vi "monitor.vi"() -> ()   [LabVIEW 2013]
uses:
  controler_custer.ctl
  <vilib>/Instr/_visa.llb/VISA Configure Serial Port (Instr).vi
panel:
  in  "Log folder":path=path "Y:/"
  in  "Sampling interval (s)":dbl=300.0
  out "DataFrontN":T1 {"Power" format="%.2g"; "Voltage" format="%.2g"; "Current" format="%.2g"; "Regulator" format="%.2g"; "Extra sensor" format="%.2g"; "Cold plate" format="%.2g"; "Set point" format="%.2g"; "Main sensor" format="%.2g"}
  in  "Input frontN":T2={"Port"="COM7", "Log file"="frontN.txt", "LogData"=TRUE}
  out "DataFrontS":T1 {"Power" format="%.2g"; "Voltage" format="%.2g"; "Current" format="%.2g"; "Regulator" format="%.2g"; "Extra sensor" format="%.2g"; "Cold plate" format="%.2g"; "Set point" format="%.2g"; "Main sensor" format="%.2g"}
  in  "Input frontS":T2={"Port"="COM6", "Log file"="frontS.txt", "LogData"=TRUE}
  out "DataBottomN":T1 {"Power" format="%.2g"; "Voltage" format="%.2g"; "Current" format="%.2g"; "Regulator" format="%.2g"; "Extra sensor" format="%.2g"; "Cold plate" format="%.2g"; "Set point" format="%.2g"; "Main sensor" format="%.2g"}
  in  "Input bottomN":T2={"Port"="COM11", "Log file"="bottomN.txt", "LogData"=TRUE}
  out "DataBottomS":T1 {"Power" format="%.2g"; "Voltage" format="%.2g"; "Current" format="%.2g"; "Regulator" format="%.2g"; "Extra sensor" format="%.2g"; "Cold plate" format="%.2g"; "Set point" format="%.2g"; "Main sensor" format="%.2g"}
  in  "Input bottomS":T2={"Port"="COM10", "Log file"="bottomS.txt", "LogData"=TRUE}
  out "DataTopN":T1 {"Power" format="%.2g"; "Voltage" format="%.2g"; "Current" format="%.2g"; "Regulator" format="%.2g"; "Extra sensor" format="%.2g"; "Cold plate" format="%.2g"; "Set point" format="%.2g"; "Main sensor" format="%.2g"}
  in  "Input topN":T3={"Port"="COM9", "Log file"="topN.txt", "logData"=TRUE}
  out "DataTopS":T1 {"Power" format="%.2g"; "Voltage" format="%.2g"; "Current" format="%.2g"; "Regulator" format="%.2g"; "Extra sensor" format="%.2g"; "Cold plate" format="%.2g"; "Set point" format="%.2g"; "Main sensor" format="%.2g"}
  in  "Input topS":T2={"Port"="COM8", "Log file"="topS.txt", "LogData"=TRUE}
  out "start time":timestamp
  in  "Connect all":bool
  in  "stop":bool
  # "Top S"
  # "Top N"
  # "Bottom S"
  # "Bottom N"
  # "Front S"
  # "Front N"
  # "Temeprature"
  # "Temeprature"
  # "Temeprature"
  # "Temeprature"
  # "Temeprature"
  # "Temeprature"
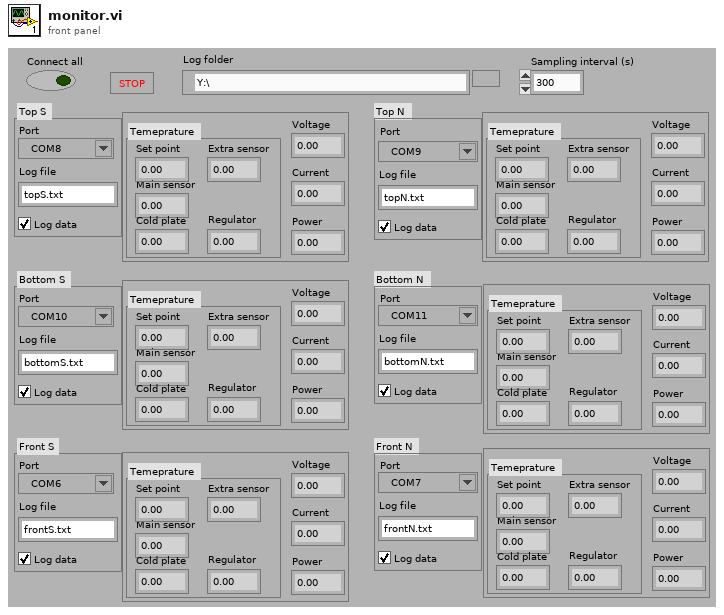
[diagram p1: front panel]
types:
  T1 = typedef "controler_custer.ctl" = cluster{"Set point":dbl, "Main sensor":dbl, "Cold plate":dbl, "Extra sensor":dbl, "Regulator":dbl, "Voltage":dbl, "Current":dbl, "Power":dbl}
  T2 = cluster{"Port":refnum<visa-resource-name>, "Log file":string, "LogData":bool}
  T3 = cluster{"Port":refnum<visa-resource-name>, "Log file":string, "logData":bool}
  T4 = cluster{"readSetPoint":string, "readT1":string, "readT2":string, "readT3":string, "readT4":string, "readV":string, "readI":string, "readPower":string}
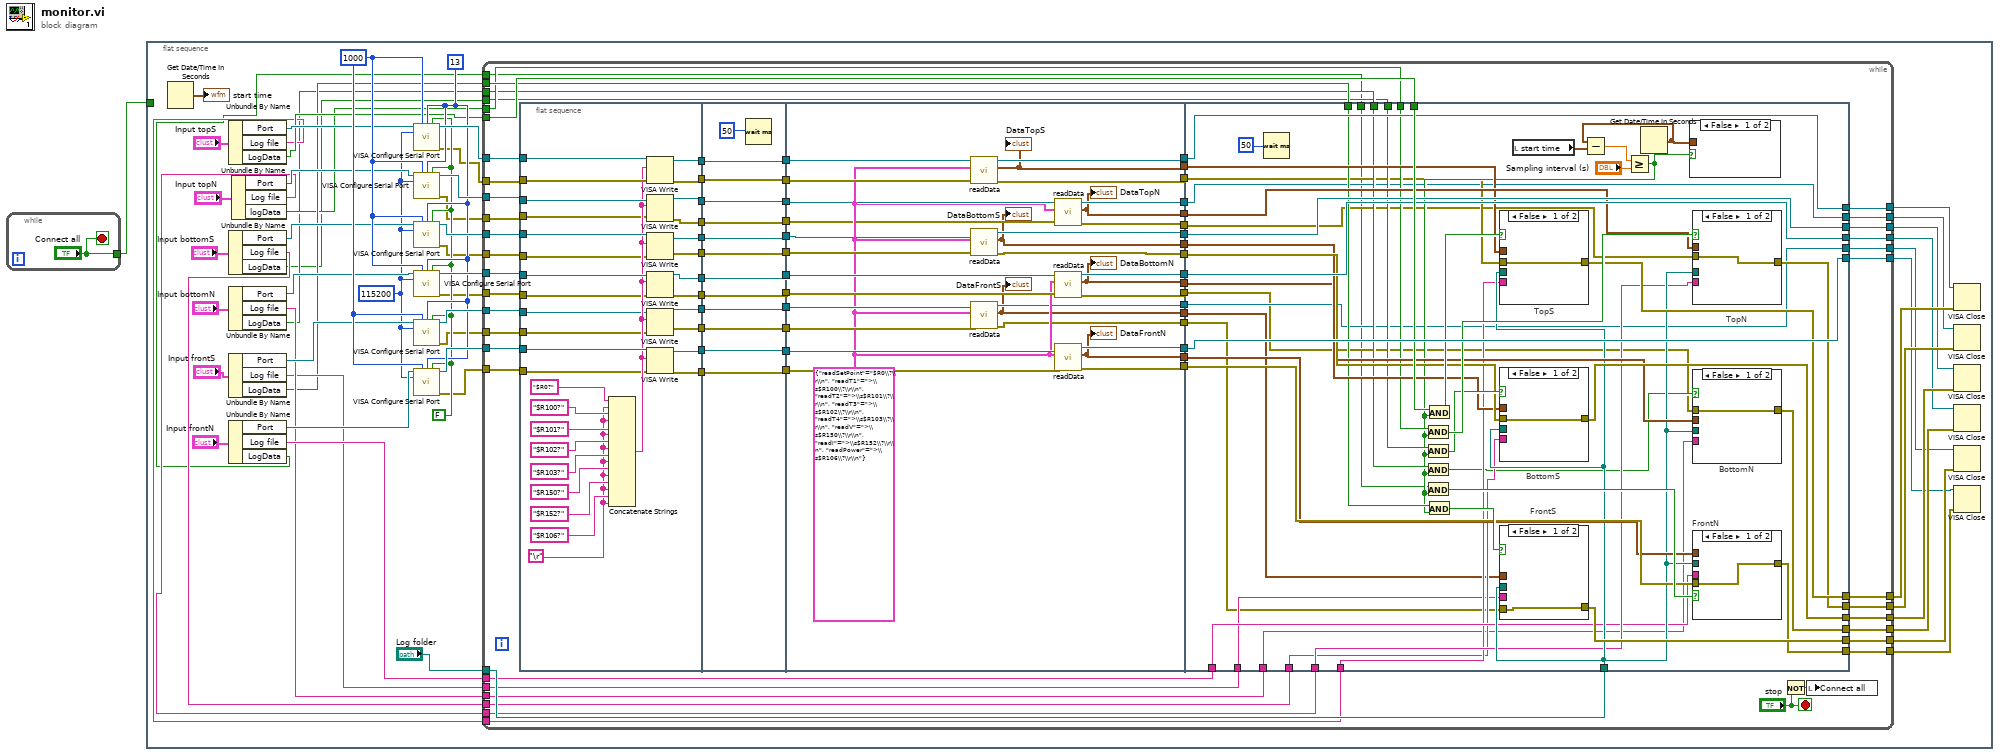
[diagram p0: block diagram]
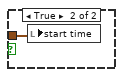
[diagram p2: hidden frame]
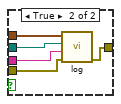
[diagram p3: hidden frame]
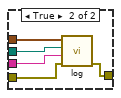
[diagram p4: hidden frame]
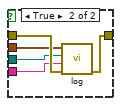
[diagram p5: hidden frame]
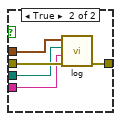
[diagram p6: hidden frame]
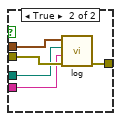
[diagram p7: hidden frame]
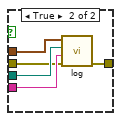
[diagram p8: hidden frame]
diagram:
  n1 = while {
    tunnel: ["Connect all"] -> w1
    stop <- "Connect all" stop-if-true
  }
  n2 = flat-sequence {
    tunnel: w1 -> [_]
    frame #0 {
      w10 = u32 115200 ("baud rate (9600)")
      w50 = u32 1000 ("timeout (10sec)")
      w48 = FALSE ("Enable Termination\nChar (T)")
      w49 = u8 13 ("termination char\n(0xA = '\\n' = LF)")
      n3 = Get Date/Time In Seconds() -> (seconds since 1Jan1904=→"start time":timestamp)
      n4 = Unbundle By Name("Input topS") -> ("Port"=w37:refnum<visa-resource-name>, "Log file"=w19:string, "LogData"=w36:bool)
      n5 = Unbundle By Name("Input bottomS") -> ("Port"=w29:refnum<visa-resource-name>, "Log file"=w18:string, "LogData"=w12:bool)
      n6 = Unbundle By Name("Input bottomN") -> ("Port"=w28:refnum<visa-resource-name>, "Log file"=w17:string, "LogData"=w13:bool)
      n7 = Unbundle By Name("Input frontS") -> ("Port"=w27:refnum<visa-resource-name>, "Log file"=w16:string, "LogData"=w15:bool)
      n8 = Unbundle By Name("Input frontN") -> ("Port"=w26:refnum<visa-resource-name>, "Log file"=w20:string, "LogData"=w11:bool)
      n9 = Unbundle By Name("Input topN") -> ("Port"=w30:refnum<visa-resource-name>, "Log file"=w21:string, "logData"=w14:bool)
      n10 = call-poly "VISA Configure Serial Port"("VISA resource name"=w37, "timeout (10sec)"=w50, "termination char\n(0xA = '\\n' = LF)"=w49, "Enable Termination\nChar (T)"=w48, "baud rate (9600)"=w10) -> ("VISA resource name out"=w56:refnum<visa-resource-name>, "error out"=w46:errorcluster)  [unwired: 9 in]
      n11 = call-poly "VISA Configure Serial Port"("VISA resource name"=w30, "timeout (10sec)"=w50, "termination char\n(0xA = '\\n' = LF)"=w49, "Enable Termination\nChar (T)"=w48, "baud rate (9600)"=w10) -> ("VISA resource name out"=w55:refnum<visa-resource-name>, "error out"=w45:errorcluster)  [unwired: 9 in]
      n12 = call-poly "VISA Configure Serial Port"("VISA resource name"=w29, "timeout (10sec)"=w50, "termination char\n(0xA = '\\n' = LF)"=w49, "Enable Termination\nChar (T)"=w48, "baud rate (9600)"=w10) -> ("VISA resource name out"=w54:refnum<visa-resource-name>, "error out"=w44:errorcluster)  [unwired: 9 in]
      n13 = call-poly "VISA Configure Serial Port"("VISA resource name"=w28, "timeout (10sec)"=w50, "termination char\n(0xA = '\\n' = LF)"=w49, "Enable Termination\nChar (T)"=w48, "baud rate (9600)"=w10) -> ("VISA resource name out"=w53:refnum<visa-resource-name>, "error out"=w43:errorcluster)  [unwired: 9 in]
      n14 = call-poly "VISA Configure Serial Port"("VISA resource name"=w27, "timeout (10sec)"=w50, "termination char\n(0xA = '\\n' = LF)"=w49, "Enable Termination\nChar (T)"=w48, "baud rate (9600)"=w10) -> ("VISA resource name out"=w52:refnum<visa-resource-name>, "error out"=w42:errorcluster)  [unwired: 9 in]
      n15 = call-poly "VISA Configure Serial Port"("VISA resource name"=w26, "timeout (10sec)"=w50, "termination char\n(0xA = '\\n' = LF)"=w49, "Enable Termination\nChar (T)"=w48, "baud rate (9600)"=w10) -> ("VISA resource name out"=w51:refnum<visa-resource-name>, "error out"=w47:errorcluster)  [unwired: 9 in]
      n16 = while {
        tunnel: w56 -> [w135]
        tunnel: w55 -> [w134]
        tunnel: w54 -> [w133]
        tunnel: w53 -> [w132]
        tunnel: w52 -> [w131]
        tunnel: w51 -> [w130]
        tunnel: [w118] -> w39
        tunnel: [w117] -> w3
        tunnel: w47 -> [w110]
        tunnel: w46 -> [w115]
        tunnel: w45 -> [w114]
        tunnel: w44 -> [w113]
        tunnel: w43 -> [w112]
        tunnel: w42 -> [w111]
        tunnel: [w97] -> w9
        tunnel: [w95] -> w40
        tunnel: w36 -> [w94]
        tunnel: [w92] -> w8
        tunnel: [w90] -> w7
        tunnel: [w88] -> w6
        tunnel: [w86] -> w5
        tunnel: [w84] -> w4
        tunnel: [w81] -> w25
        tunnel: [w78] -> w24
        tunnel: [w77] -> w23
        tunnel: "Log folder" -> [w70]
        tunnel: w21 -> [w69]
        tunnel: w20 -> [w68]
        tunnel: w19 -> [w67]
        tunnel: w18 -> [w66]
        tunnel: w17 -> [w65]
        tunnel: w16 -> [w64]
        tunnel: w15 -> [w63]
        tunnel: w14 -> [w62]
        tunnel: w13 -> [w61]
        tunnel: w12 -> [w60]
        tunnel: w11 -> [w59]
        stop <- "stop" stop-if-true
        n17 = flat-sequence {
          tunnel: w135 -> [w171]
          tunnel: w115 -> [w169]
          tunnel: [w170] -> w137
          tunnel: w134 -> [w168]
          tunnel: w133 -> [w167]
          tunnel: w132 -> [w166]
          tunnel: w131 -> [w150]
          tunnel: w130 -> [w165]
          tunnel: [w164] -> w128
          tunnel: [w163] -> w126
          tunnel: [w162] -> w125
          tunnel: [w161] -> w123
          tunnel: [w160] -> w121
          tunnel: [w159] -> w119
          tunnel: w114 -> [w149]
          tunnel: w113 -> [w148]
          tunnel: w112 -> [w147]
          tunnel: w111 -> [w146]
          tunnel: w110 -> [w145]
          tunnel: [w144] -> w108
          tunnel: [w143] -> w106
          tunnel: [w142] -> w104
          tunnel: [w141] -> w102
          tunnel: [w140] -> w100
          tunnel: w137 -> [w184]
          tunnel: [w184] -> w136
          tunnel: [w182] -> w129
          tunnel: w128 -> [w182]
          tunnel: [w181] -> w127
          tunnel: w126 -> [w181]
          tunnel: w125 -> [w173]
          tunnel: [w180] -> w124
          tunnel: w123 -> [w180]
          tunnel: [w179] -> w122
          tunnel: w121 -> [w179]
          tunnel: [w178] -> w120
          tunnel: w119 -> [w178]
          tunnel: [w177] -> w109
          tunnel: w108 -> [w177]
          tunnel: [w172] -> w107
          tunnel: w106 -> [w172]
          tunnel: [w176] -> w105
          tunnel: w104 -> [w176]
          tunnel: [w175] -> w103
          tunnel: w102 -> [w175]
          tunnel: [w174] -> w101
          tunnel: w100 -> [w174]
          tunnel: [w173] -> w99
          tunnel: w136 -> [w213]
          tunnel: w129 -> [w212]
          tunnel: w127 -> [w206]
          tunnel: w124 -> [w208]
          tunnel: w122 -> [w210]
          tunnel: w120 -> [w192]
          tunnel: [w204] -> w116
          tunnel: w109 -> [w215]
          tunnel: w107 -> [w191]
          tunnel: w105 -> [w211]
          tunnel: w103 -> [w209]
          tunnel: w101 -> [w207]
          tunnel: w99 -> [w205]
          tunnel: [w214] -> w98
          tunnel: [w202] -> w96
          tunnel: [w201] -> w93
          tunnel: [w200] -> w91
          tunnel: [w199] -> w89
          tunnel: [w198] -> w87
          tunnel: [w197] -> w85
          tunnel: [w196] -> w83
          tunnel: [w195] -> w82
          tunnel: [w194] -> w80
          tunnel: [w193] -> w79
          tunnel: [w189] -> w76
          tunnel: [w188] -> w75
          tunnel: [w187] -> w74
          tunnel: [w186] -> w73
          tunnel: [w190] -> w72
          tunnel: [w185] -> w71
          tunnel: [w242] -> w118
          tunnel: [w263] -> w117
          tunnel: w116 -> [w248]
          tunnel: w98 -> [w223]
          tunnel: [w243] -> w97
          tunnel: w96 -> [w249]
          tunnel: [w245] -> w95
          tunnel: w94 -> [w260]
          tunnel: w93 -> [w252]
          tunnel: [w252] -> w92
          tunnel: w91 -> [w221]
          tunnel: [w221] -> w90
          tunnel: w89 -> [w251]
          tunnel: [w251] -> w88
          tunnel: w87 -> [w250]
          tunnel: [w250] -> w86
          tunnel: w85 -> [w220]
          tunnel: [w220] -> w84
          tunnel: w83 -> [w263]
          tunnel: w82 -> [w218]
          tunnel: [w247] -> w81
          tunnel: w80 -> [w219]
          tunnel: [w246] -> w77
          tunnel: [w244] -> w78
          tunnel: w79 -> [w222]
          tunnel: w76 -> [w241]
          tunnel: w75 -> [w240]
          tunnel: w74 -> [w239]
          tunnel: w73 -> [w217]
          tunnel: w72 -> [w238]
          tunnel: w71 -> [w237]
          tunnel: w70 -> [w236]
          tunnel: w69 -> [w235]
          tunnel: w68 -> [w234]
          tunnel: w67 -> [w233]
          tunnel: w66 -> [w232]
          tunnel: w65 -> [w231]
          tunnel: w64 -> [w230]
          tunnel: w63 -> [w229]
          tunnel: w62 -> [w228]
          tunnel: w61 -> [w227]
          tunnel: w60 -> [w226]
          tunnel: w59 -> [w216]
          frame #0 {
            w138 = "\r"
            n18 = Concatenate Strings("$R0?" ("command"), w138, "$R100?" ("command"), w138, "$R101?" ("command"), w138, "$R102?" ("command"), w138, "$R103?" ("command"), w138, "$R150?" ("command"), w138, "$R152?" ("command"), w138, "$R106?" ("command"), w138) -> (w151:string)
            n19 = VISA Write(VISA resource name=w171, write buffer=w151, error in (no error)=w169) -> (VISA resource name out=w170:refnum<visa-resource-name>, error out=w144:errorcluster)  [unwired: 1 out]
            n20 = VISA Write(VISA resource name=w168, write buffer=w151, error in (no error)=w149) -> (VISA resource name out=w164:refnum<visa-resource-name>, error out=w143:errorcluster)  [unwired: 1 out]
            n21 = VISA Write(VISA resource name=w167, write buffer=w151, error in (no error)=w148) -> (VISA resource name out=w159:refnum<visa-resource-name>, error out=w142:errorcluster)  [unwired: 1 out]
            n22 = VISA Write(VISA resource name=w166, write buffer=w151, error in (no error)=w147) -> (VISA resource name out=w160:refnum<visa-resource-name>, error out=w141:errorcluster)  [unwired: 1 out]
            n23 = VISA Write(VISA resource name=w150, write buffer=w151, error in (no error)=w146) -> (VISA resource name out=w161:refnum<visa-resource-name>, error out=w140:errorcluster)  [unwired: 1 out]
            n24 = VISA Write(VISA resource name=w165, write buffer=w151, error in (no error)=w145) -> (VISA resource name out=w163:refnum<visa-resource-name>, error out=w162:errorcluster)  [unwired: 1 out]
          }
          frame #1 {
            n25 = Wait (ms)(milliseconds to wait=u32 50 ("attente (ms)")) -> ()  [unwired: 1 out]
          }
          frame #2 {
            w203 = T4 {"readSetPoint"="$R0\\?\\r\\n", "readT1"=">\\s$R100\\?\\r\\n", "readT2"=">\\s$R101\\?\\r\\n", "readT3"=">\\s$R102\\?\\r\\n", "readT4"=">\\s$R103\\?\\r\\n", "readV"=">\\s$R150\\?\\r\\n", "readI"=">\\s$R152\\?\\r\\n", "readPower"=">\\s$R106\\?\\r\\n"}
            n26 = call "readData.vi"("error in (no error)"=w215, "Names cluster"=w203, "VISA resource name"=w213) -> ("error out"=w214:errorcluster, "Output cluster"=w190:T1, "VISA resource name out"=w201:refnum<visa-resource-name>)  [unwired: 4 in]
            "DataTopS" <- w190
            n27 = call "readData.vi"("error in (no error)"=w211, "Names cluster"=w203, "VISA resource name"=w192) -> ("error out"=w202:errorcluster, "Output cluster"=w188:T1, "VISA resource name out"=w199:refnum<visa-resource-name>)  [unwired: 4 in]
            "DataBottomS" <- w188
            n28 = call "readData.vi"("error in (no error)"=w207, "Names cluster"=w203, "VISA resource name"=w208) -> ("error out"=w195:errorcluster, "Output cluster"=w186:T1, "VISA resource name out"=w197:refnum<visa-resource-name>)  [unwired: 4 in]
            "DataFrontS" <- w186
            n29 = call "readData.vi"("error in (no error)"=w191, "Names cluster"=w203, "VISA resource name"=w212) -> ("error out"=w193:errorcluster, "Output cluster"=w189:T1, "VISA resource name out"=w200:refnum<visa-resource-name>)  [unwired: 4 in]
            "DataTopN" <- w189
            n30 = call "readData.vi"("error in (no error)"=w209, "Names cluster"=w203, "VISA resource name"=w210) -> ("error out"=w194:errorcluster, "Output cluster"=w187:T1, "VISA resource name out"=w198:refnum<visa-resource-name>)  [unwired: 4 in]
            "DataBottomN" <- w187
            n31 = call "readData.vi"("error in (no error)"=w205, "Names cluster"=w203, "VISA resource name"=w206) -> ("error out"=w204:errorcluster, "Output cluster"=w185:T1, "VISA resource name out"=w196:refnum<visa-resource-name>)  [unwired: 4 in]
            "DataFrontN" <- w185
          }
          frame #3 {
            n32 = Wait (ms)(milliseconds to wait=u32 50 ("attente (ms)")) -> ()  [unwired: 1 out]
            n33 = local read "start time"() -> (w254:timestamp)
            n34 = Get Date/Time In Seconds() -> (seconds since 1Jan1904=w253:timestamp)
            n35 = Subtract(x=w253, y=w254) -> (x-y=w259:dbl)
            n36 = Greater Or Equal?(x=w259, y="Sampling interval (s)") -> (x >= y?=w224:bool)
            n37 = And(x=w228, y=w224) -> (x .and. y?=w258:bool)
            n38 = And(x=w226, y=w224) -> (x .and. y?=w257:bool)
            n39 = And(x=w227, y=w224) -> (x .and. y?=w225:bool)
            n40 = And(x=w216, y=w224) -> (x .and. y?=w255:bool)
            n41 = And(x=w260, y=w224) -> (x .and. y?=w261:bool)
            n42 = And(x=w229, y=w224) -> (x .and. y?=w256:bool)
            n43 = case "TopS" shown="False" w261 {
              tunnel: [w296 w301] -> w247
              tunnel: w238 -> [_ w300]
              tunnel: w236 -> [_ w299]
              tunnel: w233 -> [_ w298]
              tunnel: w223 -> [w296 w297]
              frame False {
              }
              frame True {
                n44 = call "log.vi"("error in (no error)"=w297, "FileName"=w298, "Path"=w299, "Data"=w300) -> ("error out"=w301:errorcluster)  [unwired: 6 in, 1 out]
              }
            }
            n45 = case "BottomS" shown="False" w257 {
              tunnel: w249 -> [w284 w289]
              tunnel: [w284 w288] -> w245
              tunnel: w240 -> [_ w287]
              tunnel: w236 -> [_ w286]
              tunnel: w232 -> [_ w285]
              frame False {
              }
              frame True {
                n46 = call "log.vi"("error in (no error)"=w289, "FileName"=w285, "Path"=w286, "Data"=w287) -> ("error out"=w288:errorcluster)  [unwired: 6 in, 1 out]
              }
            }
            n47 = case "FrontS" shown="False" w256 {
              tunnel: [w272 w277] -> w243
              tunnel: w217 -> [_ w276]
              tunnel: w236 -> [_ w275]
              tunnel: w230 -> [_ w274]
              tunnel: w218 -> [w272 w273]
              frame False {
              }
              frame True {
                n48 = call "log.vi"("error in (no error)"=w273, "FileName"=w274, "Path"=w275, "Data"=w276) -> ("error out"=w277:errorcluster)  [unwired: 6 in, 1 out]
              }
            }
            n49 = case shown="False" w224 {
              tunnel: w253 -> [_ w265]
              frame False {
              }
              frame True {
                n50 = local write "start time"(w265) -> ()
              }
            }
            n51 = case "TopN" shown="False" w258 {
              tunnel: w222 -> [w290 w295]
              tunnel: [w290 w294] -> w246
              tunnel: w241 -> [_ w293]
              tunnel: w236 -> [_ w292]
              tunnel: w235 -> [_ w291]
              frame False {
              }
              frame True {
                n52 = call "log.vi"("error in (no error)"=w295, "FileName"=w291, "Path"=w292, "Data"=w293) -> ("error out"=w294:errorcluster)  [unwired: 6 in, 1 out]
              }
            }
            n53 = case "BottomN" shown="False" w225 {
              tunnel: w219 -> [w278 w283]
              tunnel: [w278 w282] -> w244
              tunnel: w239 -> [_ w281]
              tunnel: w236 -> [_ w280]
              tunnel: w231 -> [_ w279]
              frame False {
              }
              frame True {
                n54 = call "log.vi"("error in (no error)"=w283, "FileName"=w279, "Path"=w280, "Data"=w281) -> ("error out"=w282:errorcluster)  [unwired: 6 in, 1 out]
              }
            }
            n55 = case "FrontN" shown="False" w255 {
              tunnel: w248 -> [w266 w271]
              tunnel: [w266 w270] -> w242
              tunnel: w237 -> [_ w269]
              tunnel: w236 -> [_ w268]
              tunnel: w234 -> [_ w267]
              frame False {
              }
              frame True {
                n56 = call "log.vi"("error in (no error)"=w271, "FileName"=w267, "Path"=w268, "Data"=w269) -> ("error out"=w270:errorcluster)  [unwired: 6 in, 1 out]
              }
            }
          }
        }
        n57 = Not(x="stop") -> (.not. x?=w57:bool)
        n58 = local write "Connect all"(w57) -> ()
      }
      n59 = VISA Close(VISA resource name=w8, error in (no error)=w25) -> ()  [unwired: 1 out]
      n60 = VISA Close(VISA resource name=w7, error in (no error)=w23) -> ()  [unwired: 1 out]
      n61 = VISA Close(VISA resource name=w6, error in (no error)=w40) -> ()  [unwired: 1 out]
      n62 = VISA Close(VISA resource name=w5, error in (no error)=w24) -> ()  [unwired: 1 out]
      n63 = VISA Close(VISA resource name=w4, error in (no error)=w9) -> ()  [unwired: 1 out]
      n64 = VISA Close(VISA resource name=w3, error in (no error)=w39) -> ()  [unwired: 1 out]
    }
  }
